vi "Update PID.vi"(8 "error in":errorcluster, 10 "ctl":cluster{"p":dbl, "i":dbl, "d":dbl}, 11 "TE Cooler in":refnum<class "TE Cooler.lvclass">) -> (0 "error out":errorcluster, 3 "TE Cooler out":refnum<class "TE Cooler.lvclass">)   [LabVIEW 2014, in "TE Cooler.lvlib" / "TE Cooler.lvclass"]
uses:
  TE Cooler.lvclass
  Controls/Command.ctl
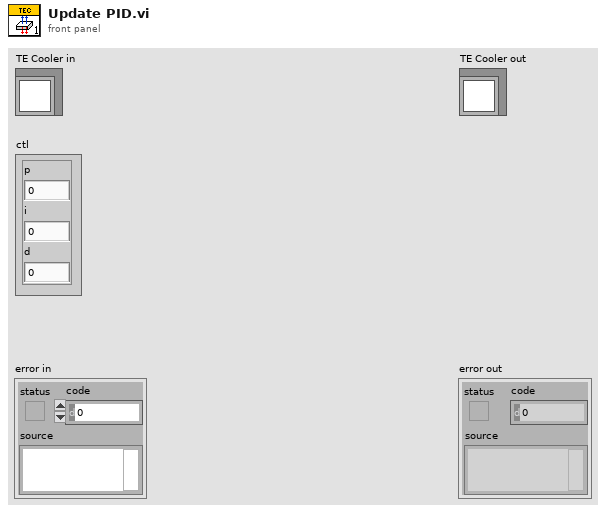
[diagram p1: front panel]
types:
  T1 = typedef "TE Cooler.lvlib/TE Cooler.lvclass/Command.ctl" = enum16{"INPUT1", "DESIRED CONTROL VALUE", "POWER OUTPUT", "ALARM STATUS", "INPUT 2", "OUTPUT CURRENT COUNTS", "ALARM TYPE", "SET TYPE DEFINE", "SENSOR TYPE", "CONTROL TYPE", "CONTROL OUTPUT POLARITY", "POWER ON/OFF", "OUTPUT SHUTDOWN IF ALARM", "FIXED DESIRED CONTROL SETTING", "PROPORTIONAL BANDWIDTH", "INTEGRAL GAIN", "DERIVATIVE GAIN", "LOW EXTERNAL SET RANGE", "HIGH EXTERNAL SET RANGE", "ALARM DEADBAND", "HIGH ALARM SETTING", "LOW ALARM SETTING", "CONTROL DEADBAND SETTING", "INPUT1 OFFSET", "INPUT2 OFFSET", "HEAT MULTIPLIER", "COOL MULTIPLIER", "OVER CURRENT COUNT COMPARE VALUE", "ALARM LATCH ENABLE", "NOT USED", "ALARM LATCH RESET", "CHOOSE SENSOR FOR ALARM FUNCTION", "CHOOSE TEMPERATURE WORKING UNITS", "EEPROM WRITE ENABLE", "OVER CURRENT CONTINUOUS", "OVER CURRENT RESTART ATTEMPTS", "JP3 DISPLAY ENABLE"}
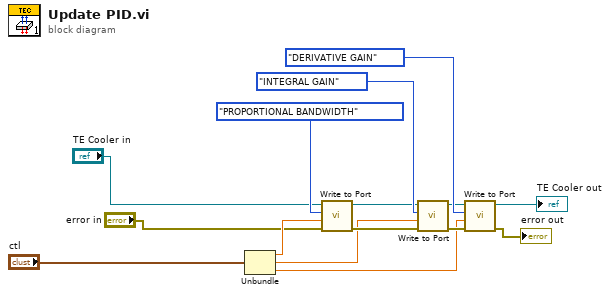
[diagram p0: block diagram]
diagram:
  n1 = Unbundle("ctl") -> ("p"=w8:dbl, "i"=w7:dbl, "d"=w6:dbl)
  n2 = call "Write to Port.vi"("error in"="error in", "Input Value"=w8, "TEC Cmd"=Command."PROPORTIONAL BANDWIDTH", "TE Cooler in"="TE Cooler in") -> ("error out"=w10:errorcluster, "TE Cooler out"=w12:refnum<class "TE Cooler.lvclass">)  [unwired: 5 in, 1 out]
  n3 = call "Write to Port.vi"("error in"=w10, "Input Value"=w7, "TEC Cmd"=Command."INTEGRAL GAIN", "TE Cooler in"=w12) -> ("error out"=w9:errorcluster, "TE Cooler out"=w11:refnum<class "TE Cooler.lvclass">)  [unwired: 5 in, 1 out]
  n4 = call "Write to Port.vi"("error in"=w9, "Input Value"=w6, "TEC Cmd"=Command."DERIVATIVE GAIN", "TE Cooler in"=w11) -> ("error out"=→"error out":errorcluster, "TE Cooler out"=→"TE Cooler out":refnum<class "TE Cooler.lvclass">)  [unwired: 5 in, 1 out]
